vi "Control Panel Sensors.vi"(9 "ArmRotatedPicture":T1, 10 "ControlPanelRotatedPicture":T1, 11 "Control Panel Motors":T3) -> (1 "Color":T2, 2 "Arm Out":bool, 3 "Arm In":bool, 4 "Control Panel Full":dbl, 5 "ArmPicture":picture, 6 "Control Panel":dbl(knob) scale=0.0..1.0, 7 "ControlPanelPicture":picture, 8 "Arm":dbl(knob) scale=0.0..1.0)   [LabVIEW 2019]
uses:
  Control Panel Motors.ctl
  Color.ctl
  Simulation Support/Rotated_Picture_TypeDef.ctl
  <vilib>/picture/pixmap.llb/Flatten Pixmap.vi
  <vilib>/picture/pictutil.llb/Create Mask.vi
  <vilib>/picture/picture.llb/Draw Flattened Pixmap.vi
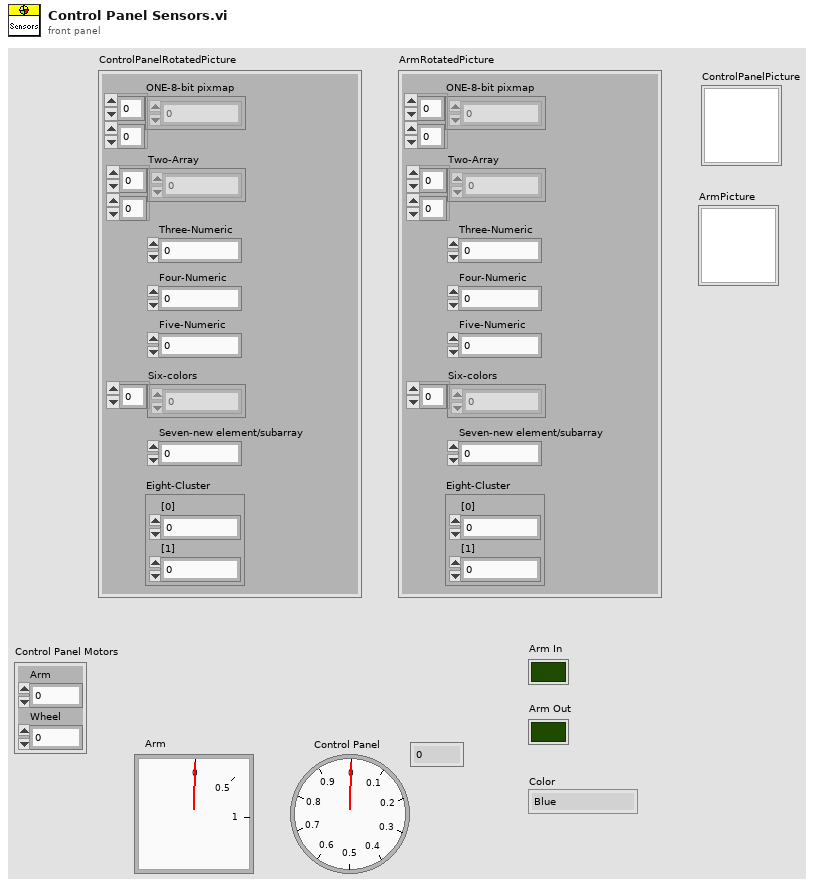
[diagram p1: front panel]
types:
  T1 = typedef "Rotated_Picture_TypeDef.ctl" = cluster{"ONE-8-bit pixmap":u8[][], "Two-Array":cdb[][], "Three-Numeric":i32, "Four-Numeric":i32, "Five-Numeric":cdb, "Six-colors":u32[], "Seven-new element/subarray":u32, "Eight-Cluster":cluster{"[0]":i32, "[1]":i32}}
  T2 = typedef "Color.ctl" = enum16{"Blue", "Green", "Red", "Yellow"}
  T3 = typedef "Control Panel Motors.ctl" = cluster{"Arm":dbl, "Wheel":dbl}
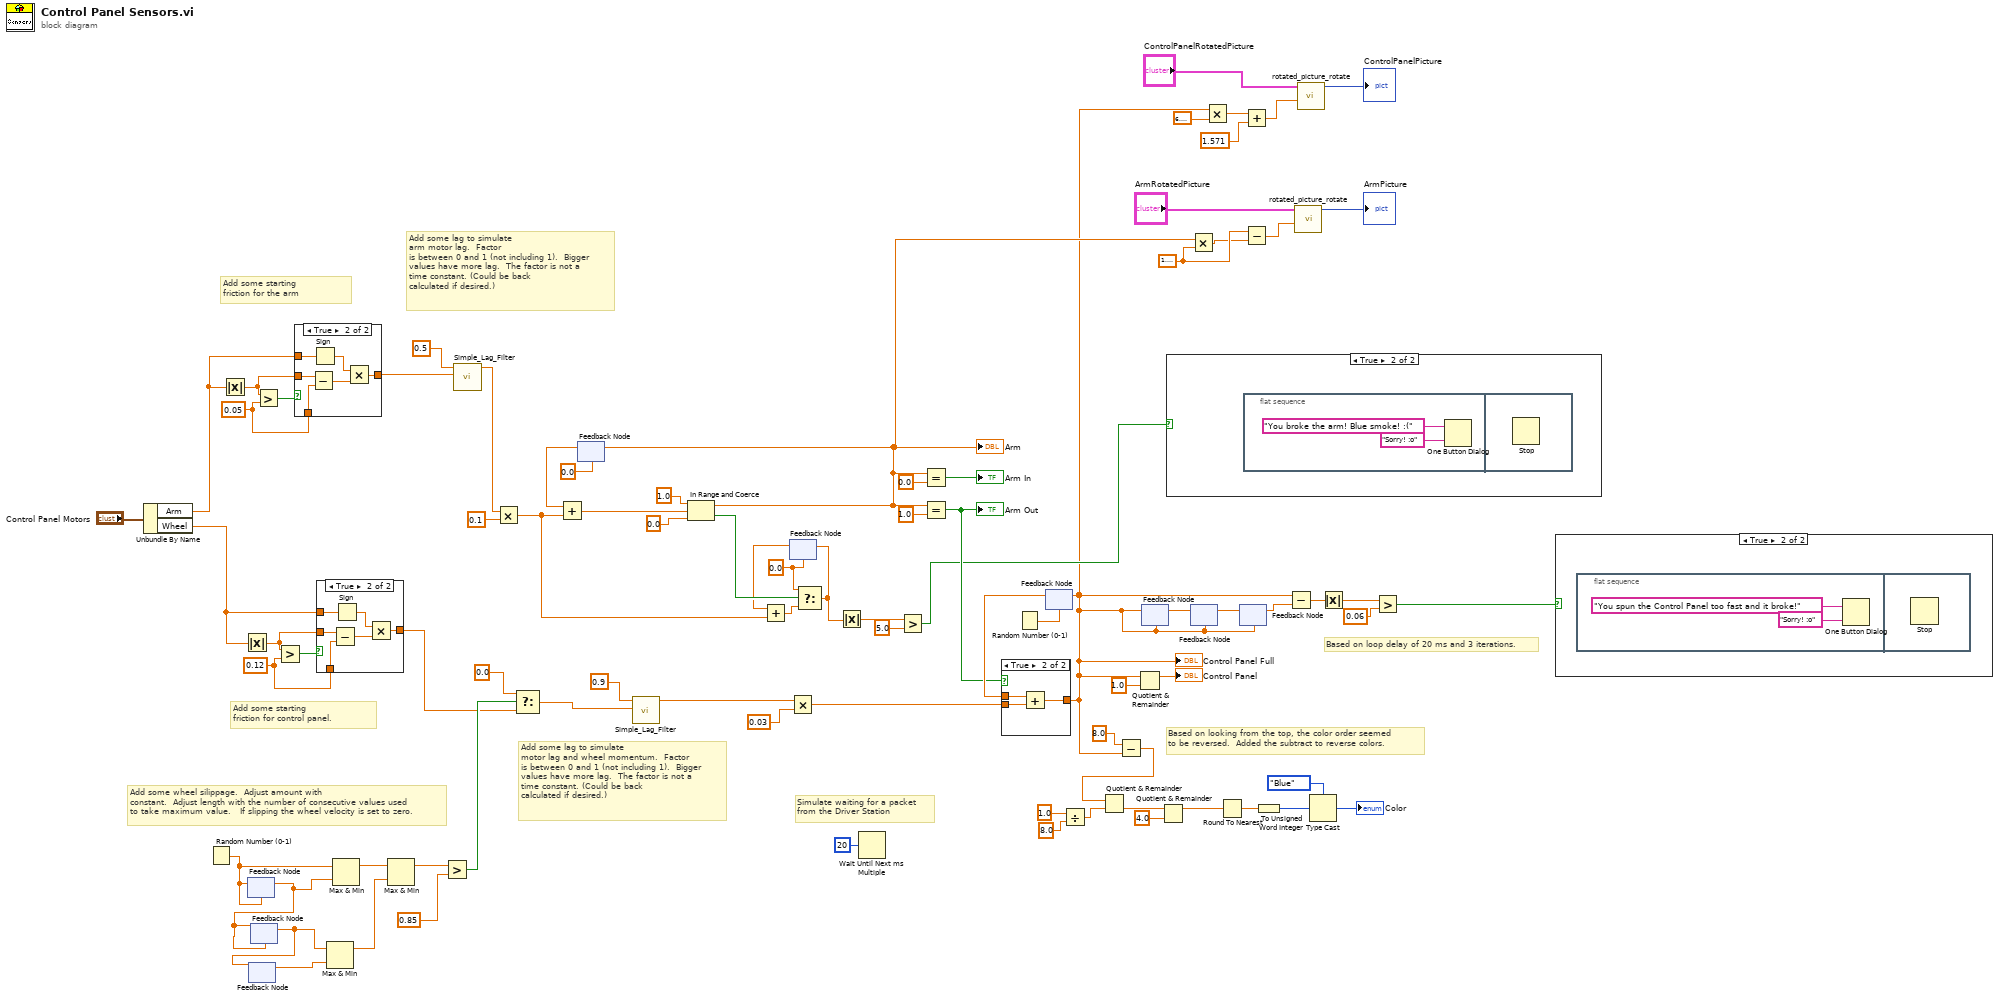
[diagram p0: block diagram]
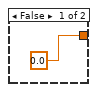
[diagram p2: hidden frame]
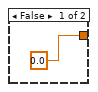
[diagram p3: hidden frame]
diagram:
  w7 = 0.05 ("y")
  w12 = 0.12 ("y")
  w30 = 1.5707963267948966
  w55 = 0.0
  # "Add some lag to simulate\narm motor lag.  Factor\nis between 0 and 1 (not including 1).  Bigger \nvalues have more lag.  The factor is not a \ntime constant. (Could be back\ncalculated if desired.)"
  # "Add some starting\nfriction for the arm"
  # "Add some starting\nfriction for control panel."
  # "Add some lag to simulate\nmotor lag and wheel momentum.  Factor\nis between 0 and 1 (not including 1).  Bigger \nvalues have more lag.  The factor is not a \ntime constant. (Could be back\ncalculated if desired.)"
  # "Add some wheel silippage.  Adjust amount with\nconstant.  Adjust length with the number of consecutive values used\nto take maximum value.   If slipping the wheel velocity is set to zero."
  # "Based on looking from the top, the color order seemed \nto be reversed.  Added the subtract to reverse colors."
  # "Based on loop delay of 20 ms and 3 iterations."
  # "Simulate waiting for a packet \nfrom the Driver Station"
  n1 = Unbundle By Name("Control Panel Motors") -> ("Arm"=w3:dbl, "Wheel"=w9:dbl)
  n2 = Random Number (0-1)() -> (number: 0 to 1=w25:dbl)
  n3 = Absolute Value(x=w3) -> (abs(x)=w6:dbl)
  n4 = Absolute Value(x=w9) -> (abs(x)=w11:dbl)
  n5 = feedback #1(w25) -> (w24:dbl)
  n6 = feedback-in #1(w25) -> ()
  n7 = feedback #2() -> (w20:dbl)  [unwired: 1 in]
  n8 = feedback #3(w24) -> (w21:dbl)
  n9 = feedback-in #2(w21) -> ()
  n10 = feedback-in #3(w24) -> ()
  n11 = Greater?(x=w6, y=w7) -> (0:w8:bool)
  n12 = Greater?(x=w11, y=w12) -> (0:w13:bool)
  n13 = case shown="True" w8 {
    tunnel: [0.0 w91] -> w2
    tunnel: w7 -> [_ w90]
    tunnel: w6 -> [_ w89]
    tunnel: w3 -> [_ w88]
    frame False {
    }
    frame True {
      n14 = Subtract(x=w89, y=w90) -> (x-y=w87:dbl)
      n15 = Sign(1:w88) -> (0:w86:dbl)
      n16 = Multiply(x=w86, y=w87) -> (x*y=w91:dbl)
    }
  }
  n17 = case shown="True" w13 {
    tunnel: [0.0 w98] -> w10
    tunnel: w12 -> [_ w97]
    tunnel: w11 -> [_ w96]
    tunnel: w9 -> [_ w95]
    frame False {
    }
    frame True {
      n18 = Subtract(x=w96, y=w97) -> (x-y=w94:dbl)
      n19 = Sign(1:w95) -> (0:w93:dbl)
      n20 = Multiply(x=w93, y=w94) -> (x*y=w98:dbl)
    }
  }
  n21 = Max & Min(x=w21, y=w20) -> (max(x,y)=w19:dbl)  [unwired: 1 out]
  n22 = Max & Min(x=w25, y=w24) -> (max(x,y)=w23:dbl)  [unwired: 1 out]
  n23 = Max & Min(x=w23, y=w19) -> (max(x,y)=w22:dbl)  [unwired: 1 out]
  n24 = Greater?(x=w22, y=0.85) -> (0:w17:bool)
  n25 = call "Simple_Lag_Filter.vi"("Input"=w2, "Lag"=0.5) -> ("Lagged Ouptut"=w4:dbl)  [unwired: 9 in]
  n26 = Multiply(x=w4, y=0.1) -> (x*y=w52:dbl)
  n27 = Select(t=0.0, s=w17, f=w10) -> (s? t:f=w16:dbl)
  n28 = feedback #4(0.0) -> (w71:dbl)
  n29 = Add(x=w71, y=w52) -> (x+y=w57:dbl)
  n30 = call "Simple_Lag_Filter.vi"("Input"=w16, "Lag"=0.9) -> ("Lagged Ouptut"=w15:dbl)  [unwired: 9 in]
  n31 = In Range and Coerce(upper limit=1.0, x=w57, lower limit=0.0) -> (coerced(x)=w31:dbl, In Range?=w56:bool)
  "Arm" <- w31
  n32 = feedback-in #4(w31) -> ()
  n33 = feedback #5(w55) -> (w53:dbl)
  n34 = Add(x=w53, y=w52) -> (x+y=w54:dbl)
  n35 = Multiply(x=w15, y=0.03) -> (x*y=w80:dbl)
  n36 = Select(t=w55, s=w56, f=w54) -> (s? t:f=w51:dbl)
  n37 = feedback-in #5(w51) -> ()
  n38 = Absolute Value(x=w51) -> (abs(x)=w49:dbl)
  n39 = Wait Until Next ms Multiple(millisecond multiple=u32 20) -> ()  [unwired: 1 out]
  n40 = Greater?(x=w49, y=5.0) -> (0:w48:bool)
  n41 = Equal?(x=w31, y=0.0) -> (x = y?=→"Arm In":bool)
  n42 = Equal?(x=w31, y=1.0) -> (x = y?=w61:bool)
  "Arm Out" <- w61
  n43 = Random Number (0-1)() -> (number: 0 to 1=w83:dbl)
  n44 = feedback #6(w83) -> (w81:dbl)
  n45 = case shown="True" w61 {
    tunnel: w81 -> [w99 w102]
    tunnel: w80 -> [_ w101]
    tunnel: [w99 w100] -> w28
    frame False {
    }
    frame True {
      n46 = Add(x=w102, y=w101) -> (x+y=w100:dbl)
    }
  }
  "Control Panel Full" <- w28
  n47 = feedback-in #6(w28) -> ()
  n48 = Divide(x=1.0, y=8.0) -> (x/y=w67:dbl)
  n49 = Subtract(x=8.0, y=w28) -> (x-y=w27:dbl)
  n50 = Quotient & Remainder(x=w27, y=w67) -> (floor(x/y)=w64:dbl)  [unwired: 1 out]
  n51 = Quotient & Remainder(x=w28, y=1.0) -> (x-y*floor(x/y)=→"Control Panel":dbl)  [unwired: 1 out]
  n52 = feedback-in #7(w28) -> ()
  n53 = feedback #7(w28) -> (w47:dbl)
  n54 = Quotient & Remainder(x=w64, y=4.0) -> (x-y*floor(x/y)=w62:dbl)  [unwired: 1 out]
  n55 = case shown="True" w48 {
    frame False {
    }
    frame True {
      n56 = flat-sequence {
        frame #0 {
          n57 = One Button Dialog(message="You broke the arm! Blue smoke! :(", button name ("OK")="Sorry! :o") -> ()  [unwired: 1 out]
        }
        frame #1 {
          n58 = Stop() -> ()  [unwired: 1 in]
        }
      }
    }
  }
  n59 = Multiply(x=w31, y=w30) -> (x*y=w29:dbl)
  n60 = feedback #8(w28) -> (w46:dbl)
  n61 = feedback-in #8(w47) -> ()
  n62 = Multiply(x=w28, y=6.283185307179586) -> (x*y=w35:dbl)
  n63 = Round To Nearest(number=w62) -> (nearest integer value=w77:dbl)
  n64 = feedback #9(w28) -> (w45:dbl)
  n65 = feedback-in #9(w46) -> ()
  n66 = Add(x=w35, y=1.571) -> (x+y=w33:dbl)
  n67 = Subtract(x=w30, y=w29) -> (x-y=w32:dbl)
  n68 = To Unsigned Word Integer(number=w77) -> (unsigned 16bit integer=w76:u16)
  n69 = Subtract(x=w28, y=w45) -> (x-y=w44:dbl)
  n70 = call "rotated_picture_rotate.vi"("Angle"=w32, "RotatedPictureInfo"="ArmRotatedPicture") -> ("new picture"=→"ArmPicture":picture)  [unwired: 9 in]
  n71 = call "rotated_picture_rotate.vi"("Angle"=w33, "RotatedPictureInfo"="ControlPanelRotatedPicture") -> ("new picture"=→"ControlPanelPicture":picture)  [unwired: 9 in]
  n72 = Type Cast(type=Color."Blue" ("Color"), x=w76) -> (*(type *) &x=→"Color":T2)
  n73 = Absolute Value(x=w44) -> (abs(x)=w43:dbl)
  n74 = Greater?(x=w43, y=0.06) -> (0:w41:bool)
  n75 = case shown="True" w41 {
    frame False {
    }
    frame True {
      n76 = flat-sequence {
        frame #0 {
          n77 = One Button Dialog(message="You spun the Control Panel too fast and it broke!", button name ("OK")="Sorry! :o") -> ()  [unwired: 1 out]
        }
        frame #1 {
          n78 = Stop() -> ()  [unwired: 1 in]
        }
      }
    }
  }
